vi "Timestamp.vi"() -> (2 "timestamp":string)   [LabVIEW 2018]
panel:
  # "ISO 8601:\nSeptember 27, 2022 at 6 p.m. is represented as 2022-09-27T18:00:00.000"
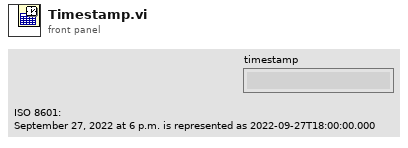
[diagram p1: front panel]
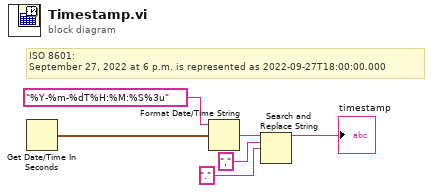
[diagram p0: block diagram]
diagram:
  # "ISO 8601:\nSeptember 27, 2022 at 6 p.m. is represented as 2022-09-27T18:00:00.000"
  n1 = Get Date/Time In Seconds() -> (seconds since 1Jan1904=w2:timestamp)
  n2 = Format Date/Time String(time format string (%c)="%Y-%m-%dT%H:%M:%S%3u", seconds (now)=w2) -> (date/time string=w5:string)  [unwired: 1 in]
  n3 = Search and Replace String(input string=w5, search string=",", replace string=".") -> (result string=→"timestamp":string)  [unwired: 5 in, 3 out]
